vi "Get image timmings.vi"(8 "error in (no error)":errorcluster, 11 "CCD in":refnum<class "CCD.lvclass">) -> (0 "error out":errorcluster, 3 "CCD out":refnum<class "CCD.lvclass">)   [LabVIEW 2018, in "CCD.lvclass"]
uses:
  CCD.lvclass
  CCD.lvclass/CCD.ctl
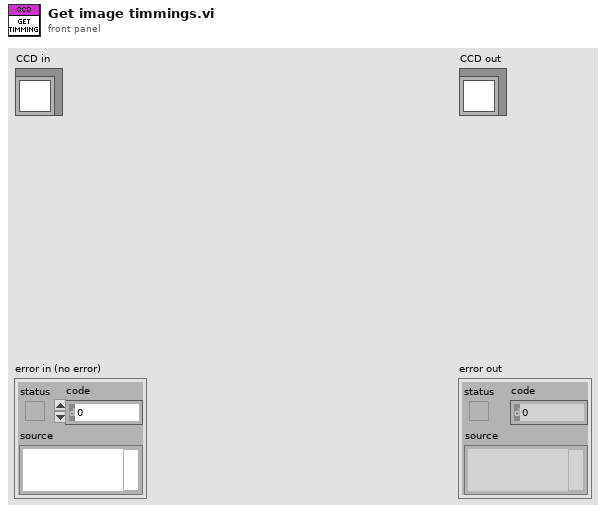
[diagram p1: front panel]
types:
  T1 = typedef "SYSTEMTIME structure typedef.ctl" = cluster{"Year":u16, "Month":u16, "DayOfWeek":u16, "Date":u16, "Hour":u16, "Minute":u16, "Second":u16, "Milliseconds":u16}
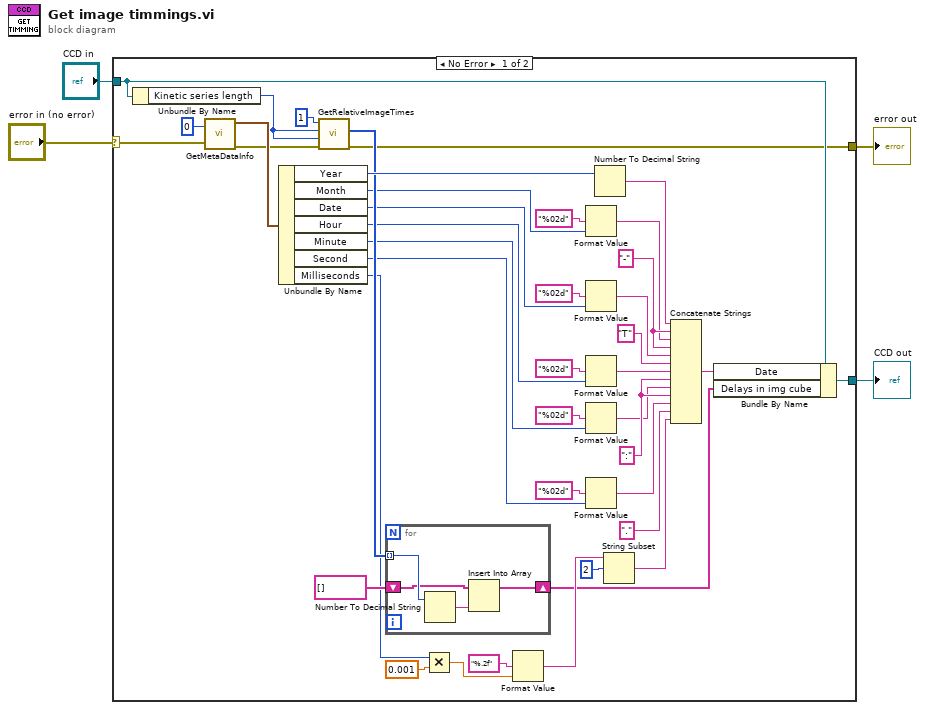
[diagram p0: block diagram]
diagram:
  n1 = case shown="No Error" "error in (no error)" {
    selector: "error in (no error)" -> [w11 w51]
    tunnel: [w5 w51] -> w2
    tunnel: [w8 w50] -> w1
    tunnel: "CCD in" -> [w9 w50]
    frame No Error {
      w37 = ":"
      w39 = "-"
      n2 = Unbundle By Name(w9) -> ("Kinetic series length"=w10:u32)
      n3 = call <userlib>:"GetMetaDataInfo.vi"("index"=0, "error in (no error)"=w11) -> ("SYSTEMTIME"=w45:T1, "error out"=w42:errorcluster)  [unwired: 2 out]
      n4 = Unbundle By Name(w45) -> ("Year"=w43:u16, "Month"=w23:u16, "Date"=w22:u16, "Hour"=w21:u16, "Minute"=w20:u16, "Second"=w19:u16, "Milliseconds"=w13:u16)
      n5 = call <userlib>:"GetRelativeImageTimes.vi"("error in (no error)"=w42, "size"=w10, "last"=w10, "first"=u32 1) -> ("error out"=w5:errorcluster, "arr"=w41:u64[])  [unwired: 5 in, 1 out]
      n6 = for {
        shift-right: [w46] -> w6
        shift-left: string[] [] -> [w47]
        tunnel: w41 -> [w49] mode=indexing
        n7 = Number To Decimal String(number=w49) -> (decimal integer string=w48:string)  [unwired: 1 in]
        n8 = Insert Into Array(array=w47, new element=w48) -> (w46:string[])  [unwired: 1 in]
      }
      n9 = Multiply(x=w13, y=0.001) -> (x*y=w18:dbl)
      n10 = Format Value(format string="%.2f", value (0)=w18) -> (output string=w17:string)  [unwired: 1 in]
      n11 = Format Value(format string="%02d", value (0)=w23) -> (output string=w32:string)  [unwired: 1 in]
      n12 = Format Value(format string="%02d", value (0)=w22) -> (output string=w30:string)  [unwired: 1 in]
      n13 = Format Value(format string="%02d", value (0)=w21) -> (output string=w28:string)  [unwired: 1 in]
      n14 = Format Value(format string="%02d", value (0)=w20) -> (output string=w26:string)  [unwired: 1 in]
      n15 = Format Value(format string="%02d", value (0)=w19) -> (output string=w24:string)  [unwired: 1 in]
      n16 = Number To Decimal String(number=w43) -> (decimal integer string=w44:string)  [unwired: 1 in]
      n17 = String Subset(string=w17, offset (0)=2) -> (substring=w12:string)  [unwired: 1 in]
      n18 = Concatenate Strings(w44, w39, w32, w39, w30, "T", w28, w37, w26, w37, w24, ".", w12) -> (w7:string)
      n19 = Bundle By Name(cluster=w9, "Date"=w7, "Delays in img cube"=w6) -> (w8:refnum<class "CCD.lvclass">)
    }
    frame Error {
    }
  }
  "error out" <- w2
  "CCD out" <- w1
